vi "Motor Decoder.vi"() -> ()   [LabVIEW 2020]
panel:
  in  "Bytes":u8[](array[numeric]) format="0x%x"
  out "Table Control":string[][](table)
  # "Motor Decoder v1.1.8"
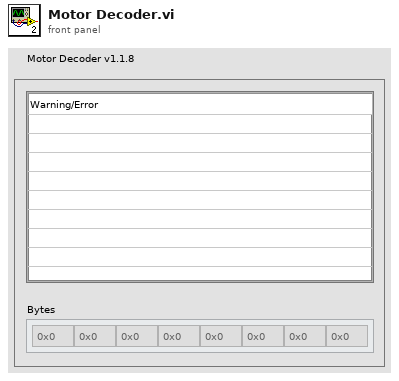
[diagram p1: front panel]
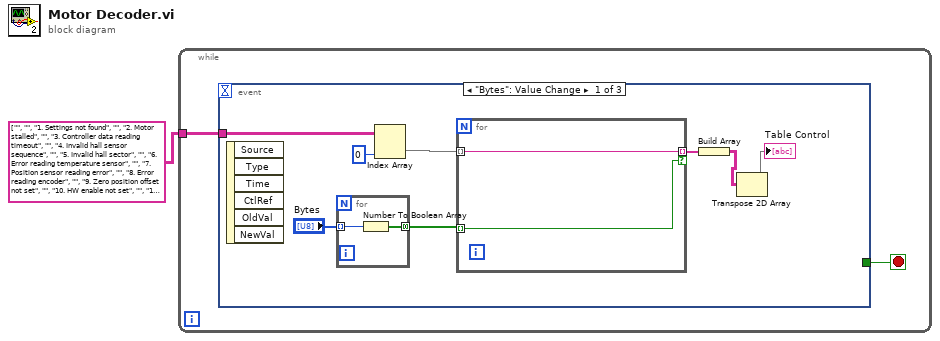
[diagram p0: block diagram]
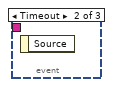
[diagram p2: hidden frame]
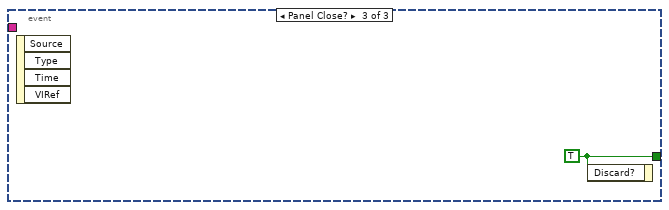
[diagram p3: hidden frame]
diagram:
  n1 = while {
    tunnel: string[][] [["", ""], ["1. Settings not found", ""], ["2. Motor stalled", ""], ["3. Controller data reading timeout", ""], ["4. Invalid hall sensor sequence", ""], ["5. Invalid hall sector", ""], ["6. Error reading temperature sensor", ""], ["7. Position sensor reading error", ""], ["8. Error reading encoder", ""], ["9. Zero position offset not set", ""], ["10. HW enable not set", ""], ["11. Error reading inverter 1 temperature", ""], ["12. Error reading inverter 2 temperature", ""], ["13. Error reading inverter 3 temperature", ""], ["14. Error reading inverter 4 temperature", ""], ["15. Error reading inverter 5 temperature", ""], ["16. Error reading inverter 6 temperature", ""], ["17. Error reading CPU temperature", "Active"], ["18. Error reading hall temperature", ""], ["19. Error reading dclink temperature", ""], ["20. Error in dclink communication", ""], ["21. Inverter 1 overcurrent", ""], ["22. Inverter 2 overcurrent", ""], ["23. Inverter 3 overcurrent", ""], ["24. Inverter 4 overcurrent", ""], ["25. Inverter 5 overcurrent", ""], ["26. Inverter 6 overcurrent", ""], ["27. DC overvoltage", ""], ["28. DC undervoltage", ""], ["29 Double CAN id on the bus", ""], ["30. CAN communication timeout", ""], ["31. Inverter 1 fault", ""], ["32. Inverter 2 fault", ""], ["33. Inverter 3 fault", ""], ["34. Inverter 4 fault", ""], ["35. Inverter 5 fault", ""], ["36. Inverter 6 fault", ""], ["37. CAN send error", ""], ["38. Lost frames on CAN bus", ""], ["39. Overspeed error", ""], ["40. CPU overloaded", ""]] ("Table Control") -> [w3]
    stop <- w2 stop-if-true
    n2 = event shown="[0] \"Bytes\": Value Change" {
      selector: _ -> [_ _ _]
      dyn-events: _ -> [_ _ _]
      timeout: _ -> [_ _ _]
      tunnel: w3 -> [w7 _ _]
      tunnel: [_ _ w16] -> w2
      event "Bytes": Value Change {
        n3 = event-data() -> ()  [unwired: 1 in, 6 out]
        n4 = for {
          tunnel: "Bytes" -> [w12] mode=indexing
          tunnel: [w13] -> w9 mode=concatenating
          n5 = Number To Boolean Array(number=w12) -> (Boolean array=w13:bool[])
        }
        n6 = Index Array(array=w7, index (col)=0 ("disabled index (col)")) -> (element=w8:string[])  [unwired: 1 in]
        n7 = for {
          tunnel: w9 -> [w14] mode=indexing
          tunnel: w8 -> [w15] mode=indexing
          tunnel: [w15] -> w11 mode=indexing if=w14
        }
        n8 = Build Array(w11) -> (w5:string[][])
        n9 = Transpose 2D Array(2D array=w5) -> (transposed array=→"Table Control":string[][])
      }
      event Timeout {
        n10 = event-data() -> ()  [unwired: 1 in, 1 out]
      }
      event Panel Close? {
        w16 = TRUE ("Discard?")
        n11 = event-data() -> ()  [unwired: 1 in, 4 out]
        n12 = event-data("Discard?"=w16) -> ()  [unwired: 1 in, 1 out]
      }
    }
  }
